vi "find centroid.vi"(0 "LVImagePtrSrc":string, 1 "LVLineWidthSrc":i32, 2 "LVImagePtrDst":string, 3 "LVLineWidthDst":i32, 4 "LVWidth":i32, 5 "LVHeight":i32, 6 "BinThresh":i32, 7 "error in (no error)":errorcluster, 8 "Esize":i32, 9 "centroid":cluster{}) -> (19 "centroid out":cluster{}, 20 "LVImagePtrSrc out":string, 21 "function return":i32, 22 "LVImagePtrDst out":string, 27 "error out":errorcluster)   [LabVIEW 2012, in "find_fish_position.lvlib"]
doc: "int FIND_FISH_POSITION_DLL find_centroid(char* LVImagePtrSrc, int LVLineWidthSrc,\n char* LVImagePtrDst, int LVLineWidthDst,\n int LVWidth, int LVHeight, int BinThresh, int Esize, Point *centroid);"
uses:
  find_fish_position.lvlib
  find_fish_position.dll
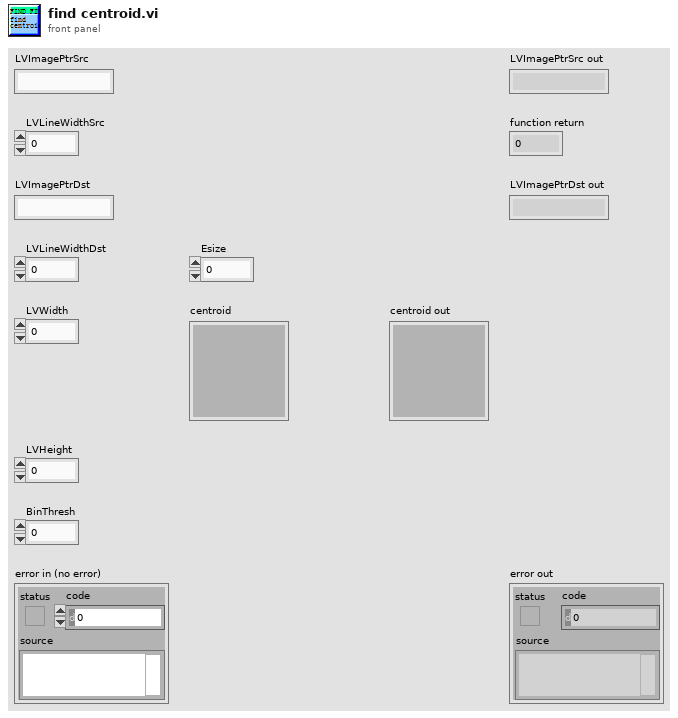
[diagram p1: front panel]
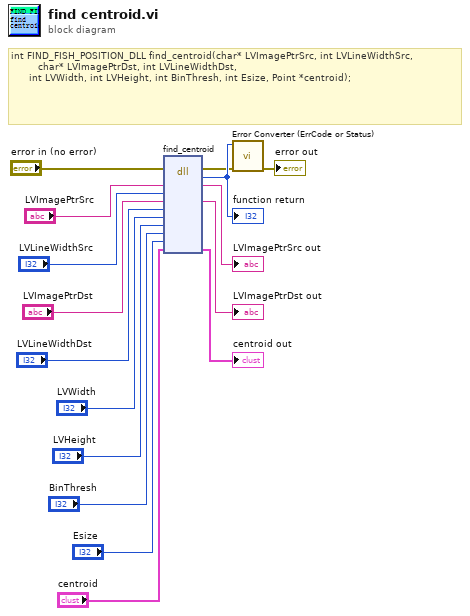
[diagram p0: block diagram]
diagram:
  # "int FIND_FISH_POSITION_DLL find_centroid(char* LVImagePtrSrc, int LVLineWidthSrc,\n\t\t\t      char* LVImagePtrDst, int LVLineWidthDst,\n\t\t\t\t  int LVWidth, int LVHeight, int BinThresh, int Esize, Point *centroid);"
  n1 = dll-call lib="C:/Users/quan/workspace/fish tracking dll/labview/find_fish_position.*" fn="find_centroid"(error in="error in (no error)", "LVImagePtrSrc"="LVImagePtrSrc", "LVLineWidthSrc"="LVLineWidthSrc", "LVImagePtrDst"="LVImagePtrDst", "LVLineWidthDst"="LVLineWidthDst", "LVWidth"="LVWidth", "LVHeight"="LVHeight", "BinThresh"="BinThresh", "Esize"="Esize", "centroid"="centroid") -> (error out=w2:errorcluster, w16:i32, "LVImagePtrSrc"=→"LVImagePtrSrc out":string, "LVImagePtrDst"=→"LVImagePtrDst out":string, "centroid"=→"centroid out":cluster{})  [unwired: 8 in, 1 out]
  "function return" <- w16
  n2 = call "Error Converter (ErrCode or Status).vi"("error in (no error)"=w2, "error code"=w16) -> ("error out"=→"error out":errorcluster)  [unwired: 9 in]
